vi "2D Gaussian - Fit Testing.vi"() -> ()   [LabVIEW 2016]
uses:
  2D Gaussian - Type Defs/2D Gaussian - Best Fit Parameters.ctl
panel:
  out "Fit Results":T1
  in  "Columns (X)":i32
  out "Generated":dbl[][](graph)
  in  "Rows (Y)":i32
  in  "Parameters":dbl[](array[numeric])
  # "When you generate a 2D Gaussian of type DOUBLE with a small amplitude and then\nconvert to U16 you lose all the decimal places and wont get a very good fit."
  # "Amplitude\nX Position\nY Position\nX Width\nY Width\nOffset"
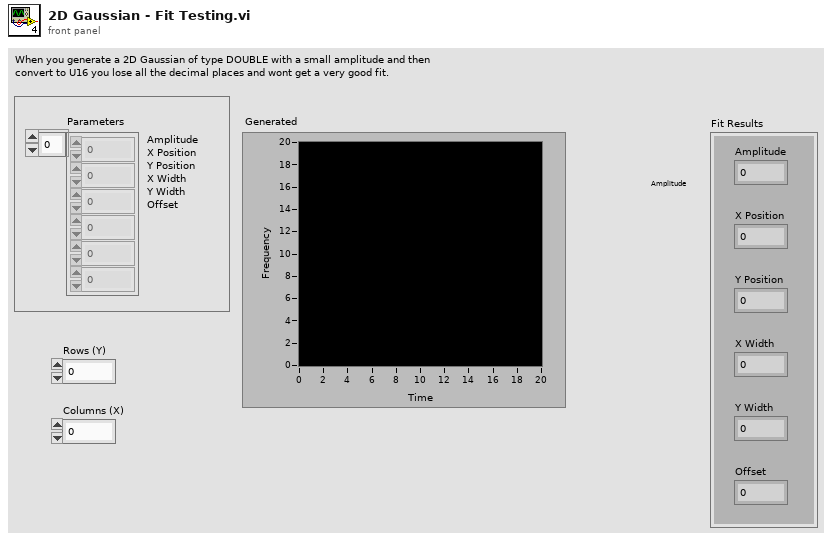
[diagram p1: front panel]
types:
  T1 = typedef "2D Gaussian - Best Fit Parameters.ctl" = cluster{"Amplitude":dbl, "X Position":dbl, "Y Position":dbl, "X Width":dbl, "Y Width":dbl, "Offset":dbl}
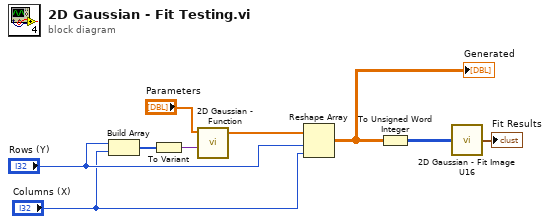
[diagram p0: block diagram]
diagram:
  n1 = Build Array("Rows (Y)", "Columns (X)") -> (w4:i32[])
  n2 = To Variant(anything=w4) -> (Variant=w3:variant)
  n3 = call "2D Gaussian - Function.vi"("data"=w3, "a"="Parameters") -> ("f(X,a)"=w8:dbl[])  [unwired: 2 in, 2 out]
  n4 = Reshape Array(w8, "Rows (Y)", "Columns (X)") -> (w7:dbl[][])
  "Generated" <- w7
  n5 = To Unsigned Word Integer(number=w7) -> (unsigned 16bit integer=w2:u16[][])
  n6 = call "2D Gaussian - Fit Image U16.vi"("Image In (U16)"=w2) -> ("Best Fit Params"=→"Fit Results":T1)  [unwired: 14 in]
